vi "Scope_5772.vi"() -> ()   [LabVIEW 2013]
uses:
  <vilib>/rvi/interface/nirviReadWriteControl/nirviReadWriteControl.xnode
  <vilib>/rvi/errors/niLvFpgaAdjustHostInterfaceError.vi
  <vilib>/rvi/interface/nirviCloseFPGA/nirviCloseFPGA.xnode
  FPGA/DataMode.ctl
  <vilib>/rvi/interface/nirviOpenFPGA/nirviOpenFPGA.xnode
  <vilib>/Utility/error.llb/Error Cluster From Error Code.vi
  NiFpgaLv.dll
  <vilib>/rvi/interface/Simulation/niFpgaSimulationCallBeginRW.vi
  Host/Utilities/Ticker/Ticker.lvclass
  Host/Config/FPGAref.ctl
  Host/Scope/controls/ScopeMode.ctl
  FPGA Bitfiles/mixer_FPGATarget_FPGAmain5772_HJBBnI0CKw8.lvbitx
  <vilib>/FPGAPlugInAG/PXIe-7975R/niLvFpga_Open_PXIe-7975R.vi
  <vilib>/rvi/interface/common/dynamic/niFpgaDynamicAddResources.vi
  <vilib>/FPGAPlugInAG/Dynamic/niLvFpga_Close_Dynamic.vi
  <vilib>/userdefined/High Color/nirio_resource_hc.ctl
  <vilib>/Analysis/4window.llb/windowTd.ctl
  <vilib>/Analysis/NI_AALPro.lvlib
  Host/Scope/controls/power_spectrum_unit.ctl
panel:
  in  "Zoom freq X":bool
  in  "Zoom freq Y":bool
  in  "Zoom time Y":bool
  in  "Zoom time X":bool
  in  "Unit":T1
  in  "Window":T2=1 items=["Rectangle"=0, "Hanning"=1, "Hamming"=2, "Blackman-Harris"=3, "Exact Blackman"=4, "Blackman"=5, "Flat Top"=6, "4 Term B-Harris "=7, "7 Term B-Harris"=8, "Low Sidelobe"=9, "Blackman Nuttall"=11, "Triangle"=30, "Bartlett-Hanning"=31, "Bohman"=32, "Parzen"=33, "Welch"=34, "Kaiser"=60, "Dolph-Chebyshev"=61, "Gaussian"=62]
  in  "Samples to aqcuire":u32
  in  "Mode":T3
  in  "Mixer freq [MHz]":dbl
  in  "Phase offset (deg)":dbl
  in  "Fequency [MHz]":dbl
  in  "Ch1":bool
  in  "Ch0":bool
  out "freqdata":cluster{"f0":dbl, "df":dbl, "magnitude":dbl[]}[](graph)
  out "Timedata":dbl[][](graph)
  in  "Rumode":bool
  in  "Singleshot":bool
  in  "Ch1 Q":bool
  in  "Ch1 I":bool
  in  "Ch0 Q":bool
  in  "Ch0 I":bool
  out "error IO":errorcluster
  in  "stop":bool
  in  "resource name":T4="RIO0"
  out "Clocking Option Configured?":bool
  out "Configured?":bool
  # "Auto Zoom"
  # "Auto Zoom"
  # "FFT"
  # "Time domain"
  # "FPGA setup"
  # "Simulated data"
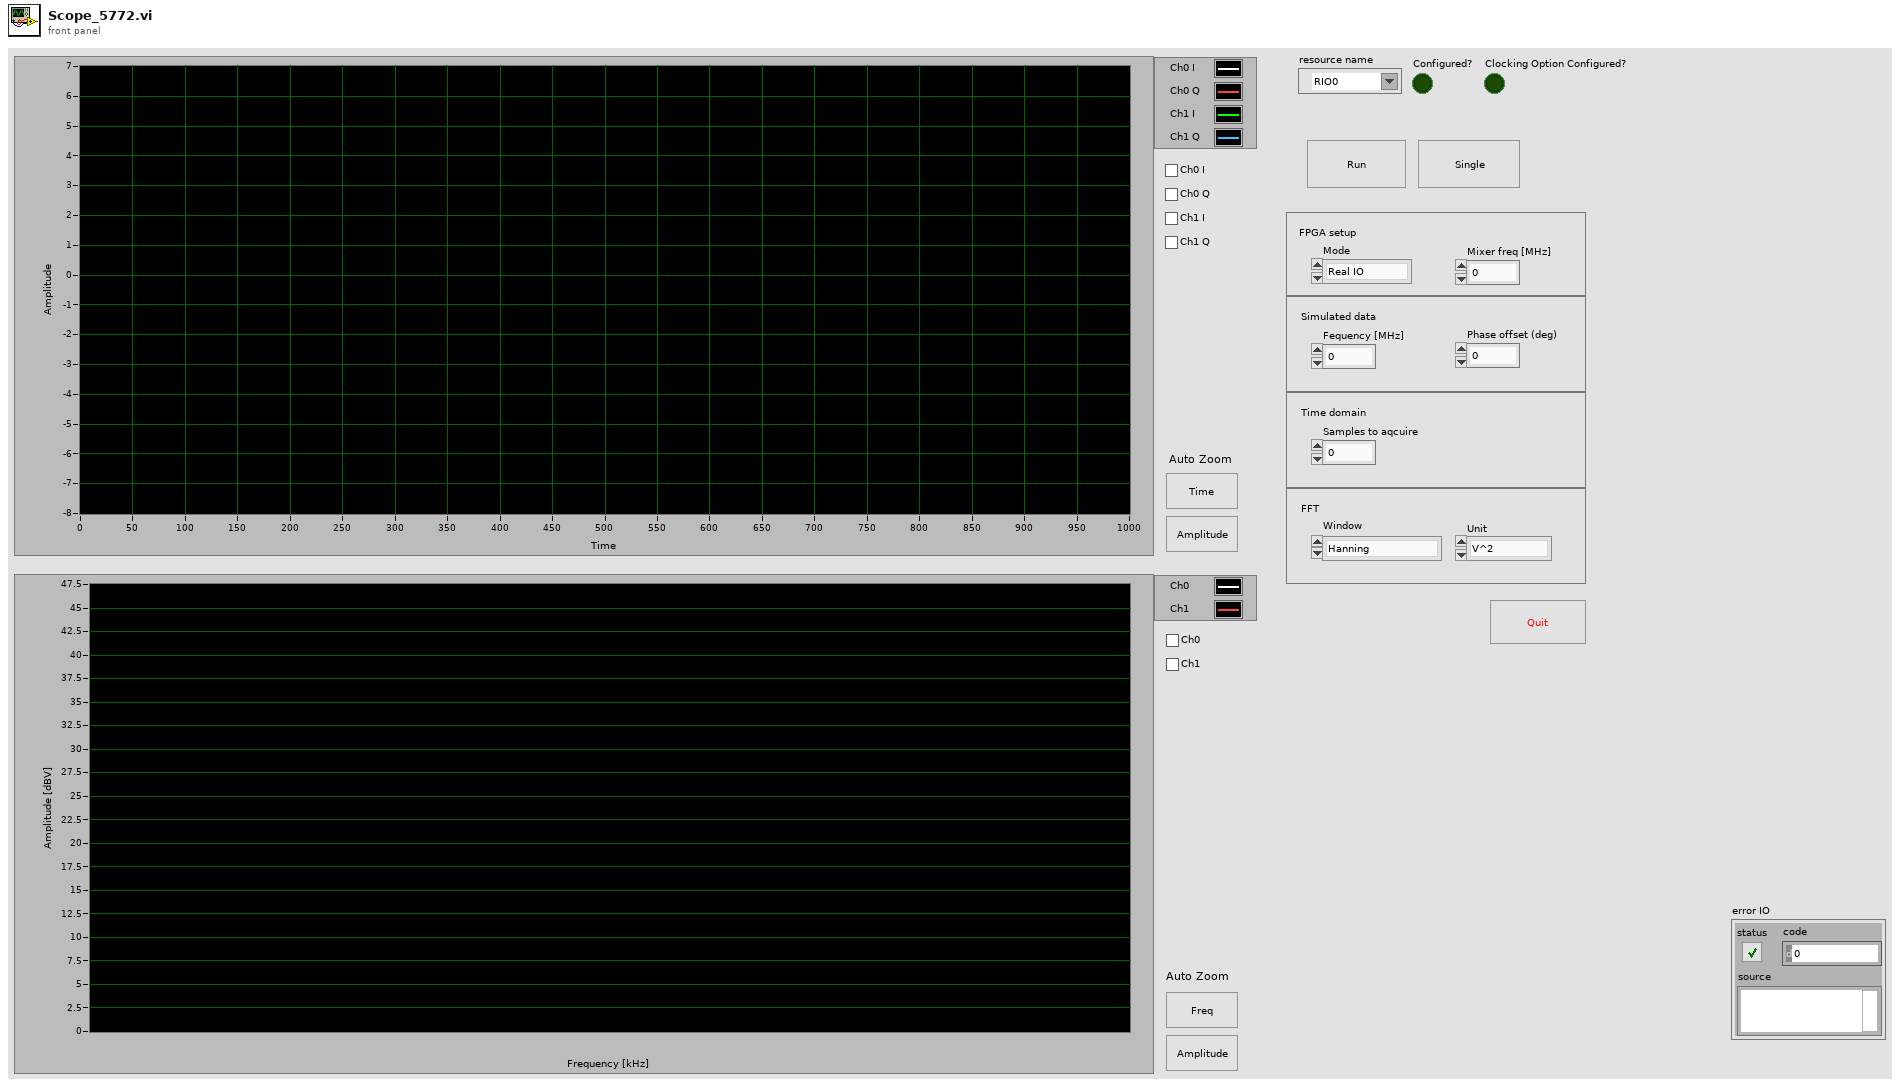
[diagram p1: front panel]
types:
  T1 = typedef "power_spectrum_unit.ctl" = enum16{"V^2", "V", "dBV"}
  T2 = typedef "NI_AALPro.lvlib/windowTd.ctl" = u32
  T3 = typedef "DataMode.ctl" = enum16{"Real IO", "Simulated"}
  T4 = typedef "nirio_resource_hc.ctl" = tag
  T5 = enum8{"Internal Clock PLL Off", "Internal Clock PLL On (REF IN)", "External Clock (CLK_IN)", "Internal Clock PLL On (IoModSyncClk)"}
  T6 = typedef "FPGAref.ctl" = refnum<k20>
  T7 = typedef "scope_params.ctl" = cluster{"scope mode":T8, "ticker":refnum<class "Ticker.lvclass">, "5160 samples per trigger":u32, "FPGA ref":T6, "P2P params":T9, "data mode":T3, "5782 samples per record":u32, "Chart length":i32}
  T8 = typedef "ScopeMode.ctl" = enum16{"Stopped", "Single", "Running", "Continuous"}
  T9 = typedef "P2P params.ctl" = cluster{"instrument handle":refnum<k15>, "stream session":refnum<k20>, "scale":cluster{"offset":dbl, "gain":dbl, "reserved 1":dbl, "reserved 2":dbl}, "actual sample rate":dbl, "Trigger":T10, "SCOPE Resource":refnum<k15>, "input impedance":u32}
  T10 = typedef "trigger_source.ctl" = enum16{"PFI 0", "PFI 1", "Software"}
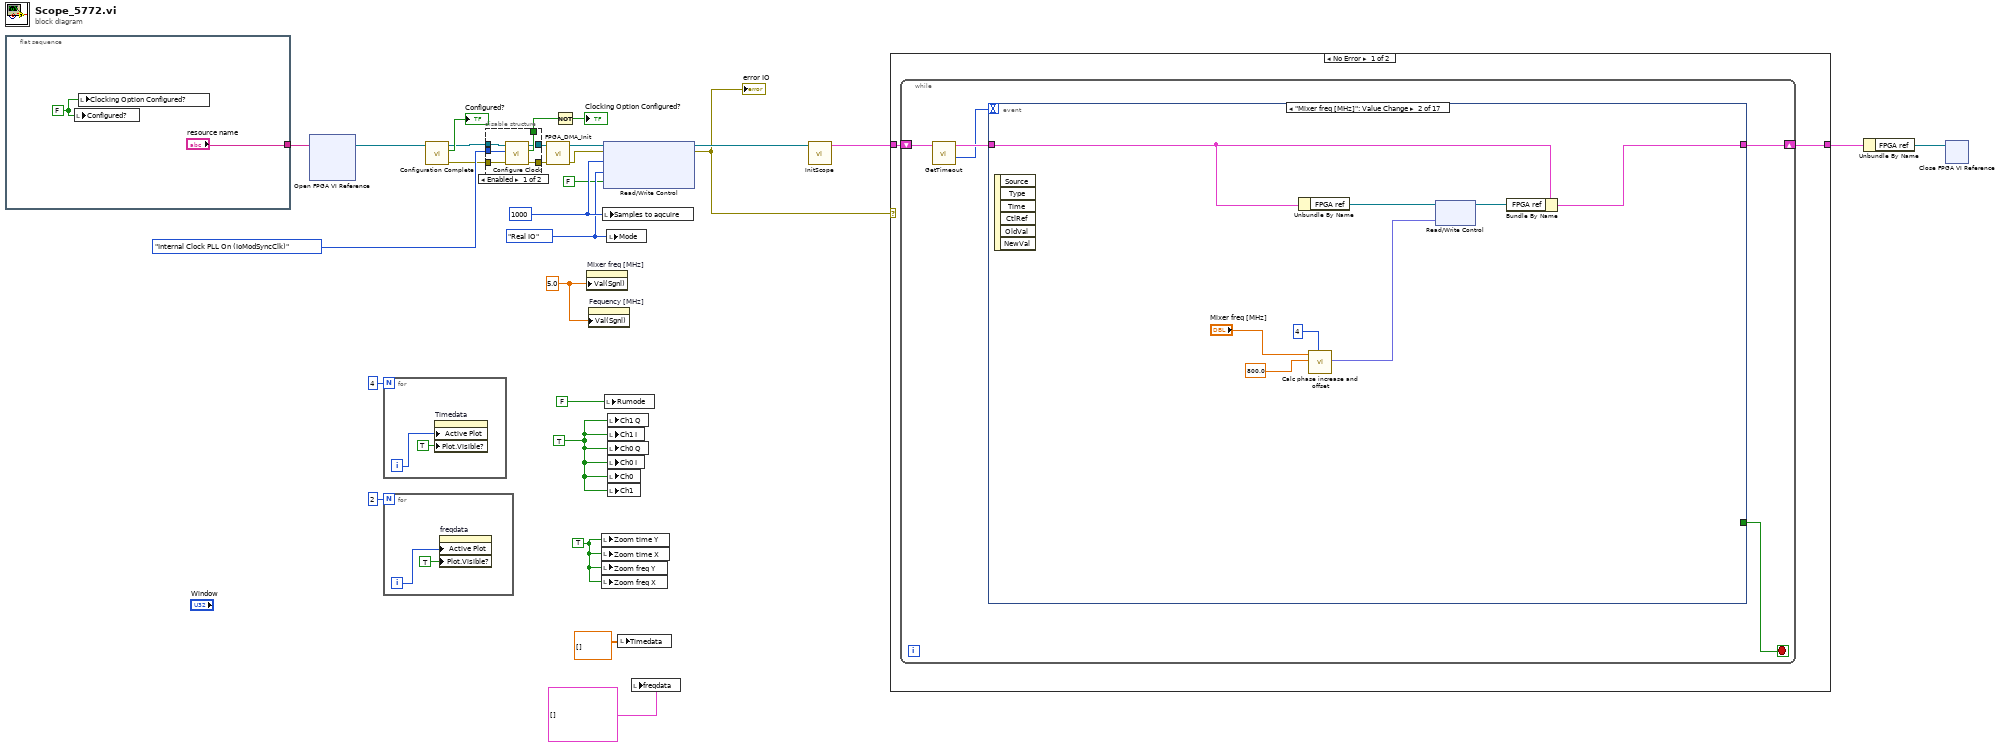
[diagram p0: block diagram]
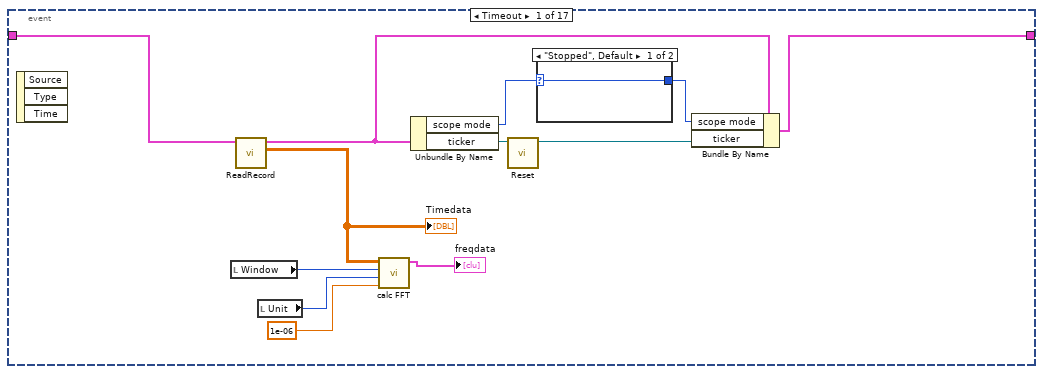
[diagram p3: hidden frame]
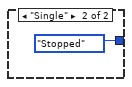
[diagram p4: hidden frame]
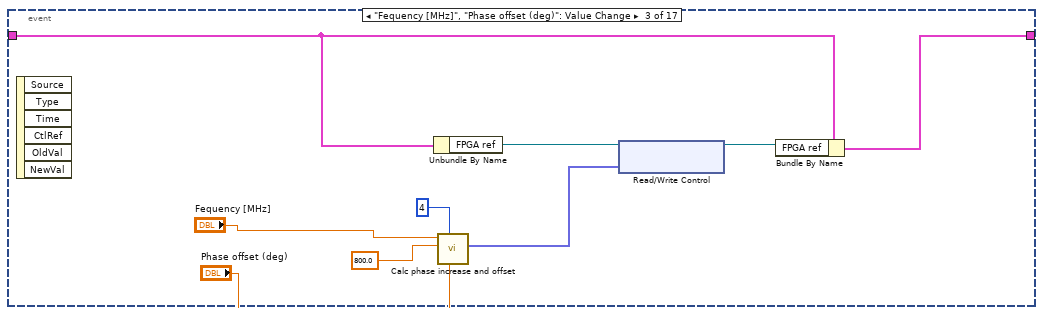
[diagram p5: hidden frame]
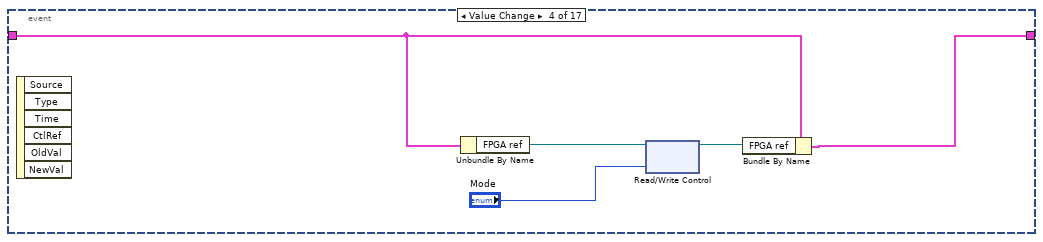
[diagram p6: hidden frame]
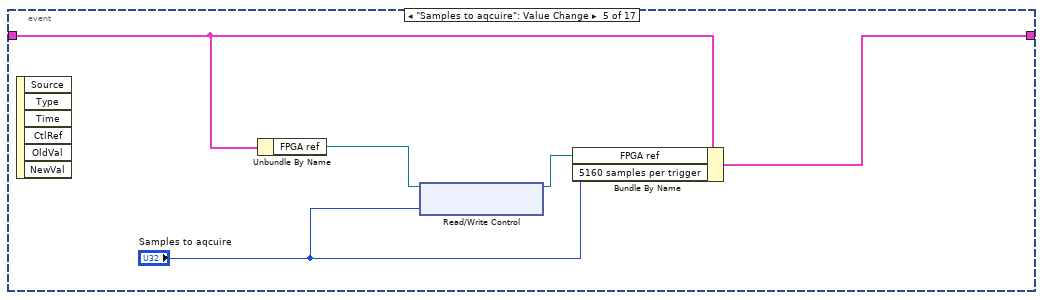
[diagram p7: hidden frame]
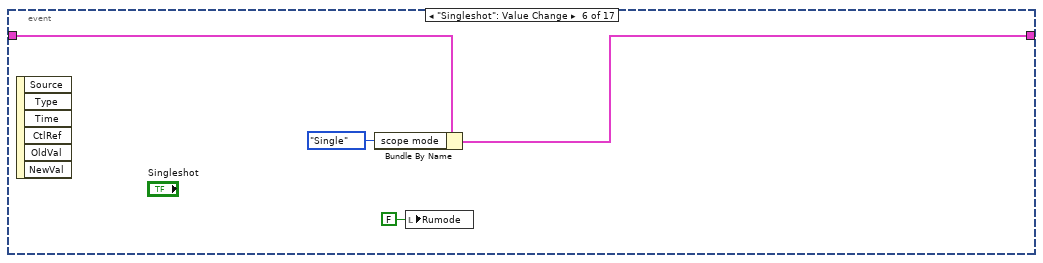
[diagram p8: hidden frame]
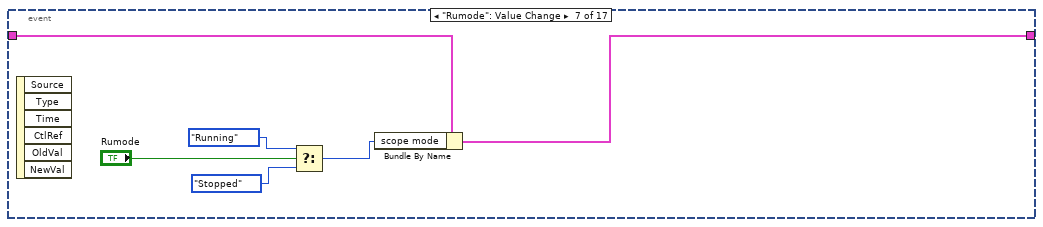
[diagram p9: hidden frame]
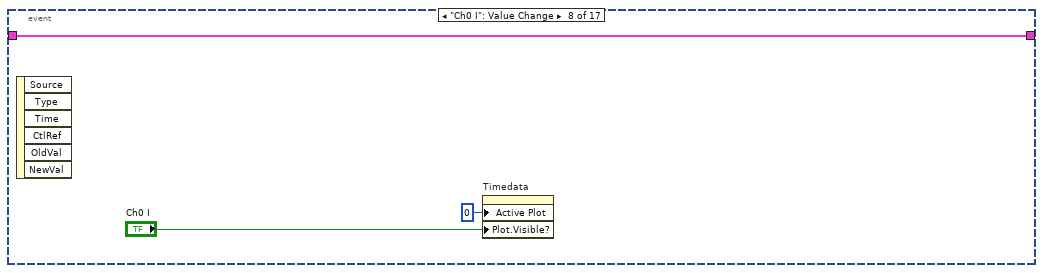
[diagram p10: hidden frame]
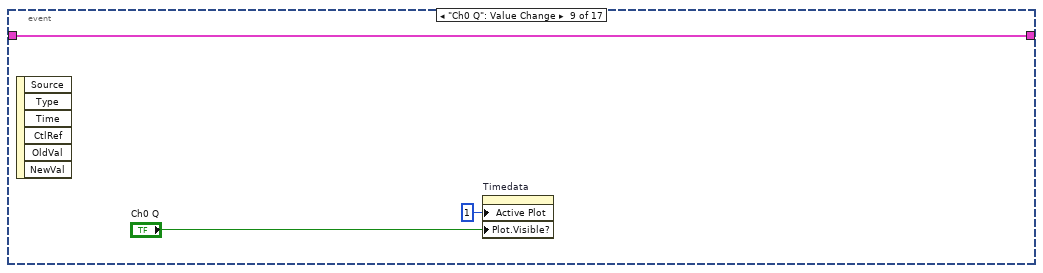
[diagram p11: hidden frame]
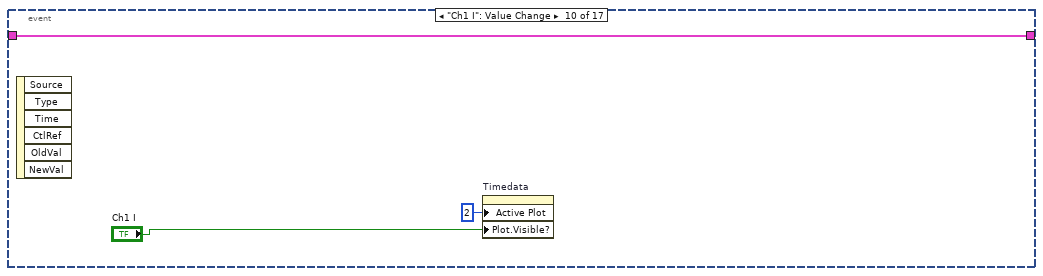
[diagram p12: hidden frame]
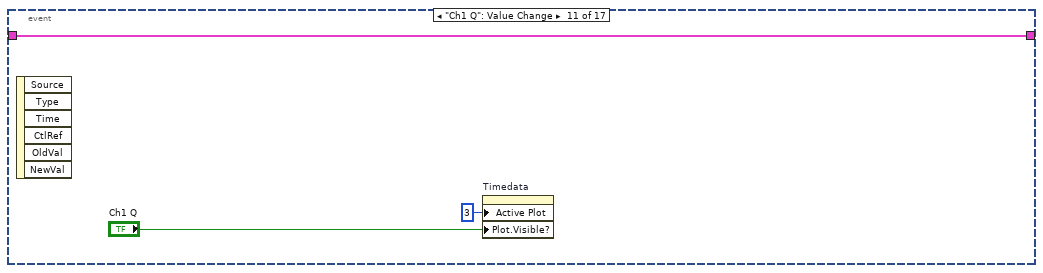
[diagram p13: hidden frame]
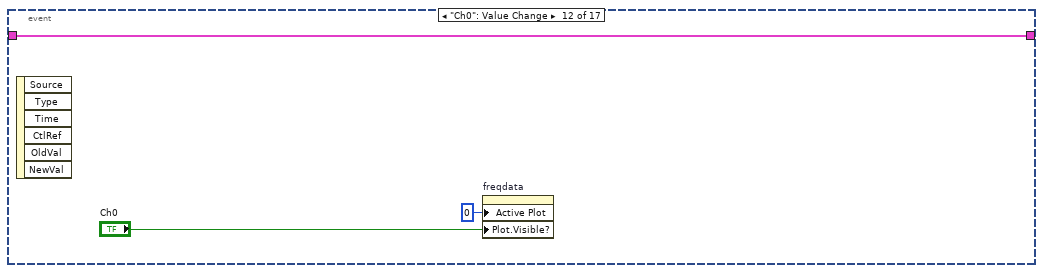
[diagram p14: hidden frame]
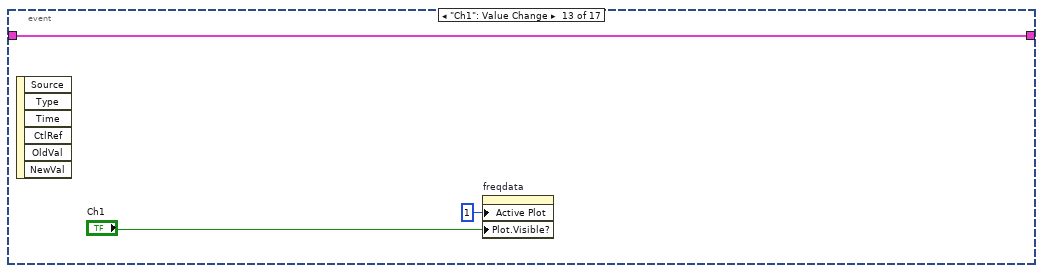
[diagram p15: hidden frame]
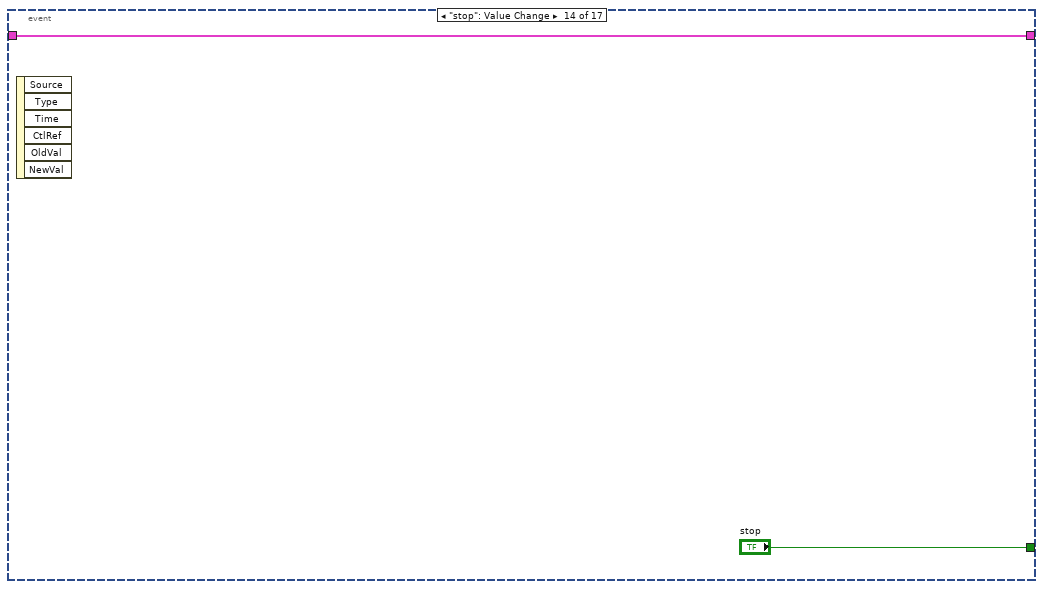
[diagram p16: hidden frame]
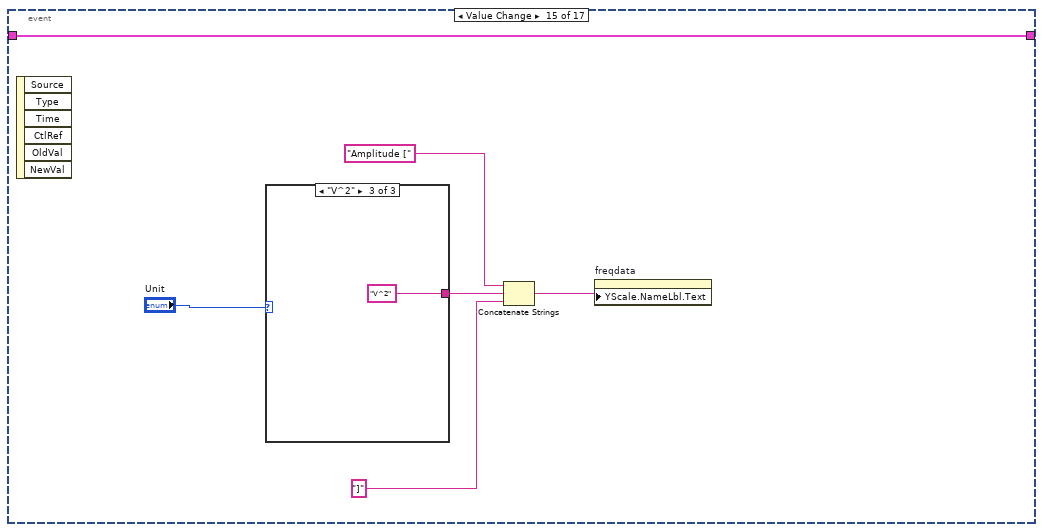
[diagram p17: hidden frame]
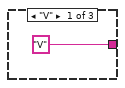
[diagram p18: hidden frame]
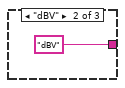
[diagram p19: hidden frame]
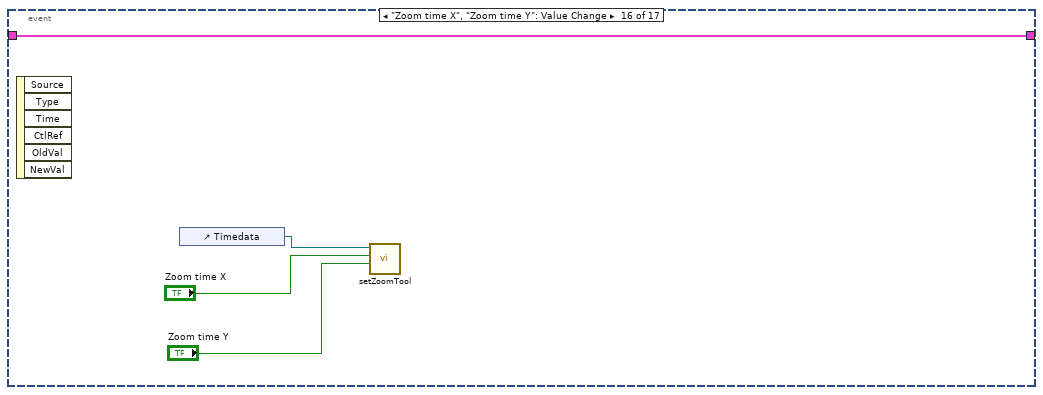
[diagram p20: hidden frame]
diagram:
  w1 = TRUE ("Rumode")
  w2 = TRUE ("Rumode")
  w6 = 5.0 ("Mixer requency [MHz]")
  w21 = DataMode."Real IO" ("Mode")
  w22 = u32 1000 ("Samples to aqcuire")
  n1 = flat-sequence {
    tunnel: ["resource name"] -> w16
    frame #0 {
      w29 = FALSE ("Trigger Acquisition")
      n2 = local write "Configured?"(w29) -> ()
      n3 = local write "Clocking Option Configured?"(w29) -> ()
    }
  }
  n4 = xnode "Open FPGA VI Reference"("resource name"=w16) -> ("FPGA VI Reference Out"=w11:refnum<k20>)  [unwired: 1 in, 1 out]
  n5 = for {
    N: 4 -> [_]
    i -> [w32]
    n6 = property on="Timedata" class="WFGraph (strict)"("Active Plot"=w32, "Plot.Visible?"=TRUE ("Plot.Visible")) -> ()  [unwired: 2 in, 2 out]
  }
  n7 = for {
    N: 2 -> [_]
    i -> [w33]
    n8 = property on="freqdata" class="WFGraph (strict)"("Active Plot"=w33, "Plot.Visible?"=TRUE ("Plot.Visible")) -> ()  [unwired: 2 in, 2 out]
  }
  n9 = call "Configuration Complete.vi"("FPGA VI Reference in"=w11) -> ("error out"=w19:errorcluster, "Configured?"=→"Configured?":bool, "FPGA VI Reference Out"=w9:T6)  [unwired: 8 in]
  n10 = disable-structure shown="Enabled" {
    disable-tunnel: [w40 _] -> w26
    disable-tunnel: T5."Internal Clock PLL On (IoModSyncClk)" ("Clock Source") -> [w39 _]
    disable-tunnel: [w38 w42] -> w24
    disable-tunnel: w19 -> [w37 w41]
    disable-tunnel: [w36 w41] -> w18
    disable-tunnel: w9 -> [w35 _]
    frame Enabled {
      n11 = call "Configure Clock.vi"("error in"=w37, "Clock Source"=w39, "FPGA VI Reference in"=w35) -> ("error out"=w36:errorcluster, "Configuration Error"=w40:bool, "FPGA VI Reference Out"=w38:T6)  [unwired: 6 in]
    }
    frame Disabled {
    }
  }
  n12 = call "FPGA_DMA_Init.vi"("error in (no error)"=w18, "FPGA VI Reference"=w24) -> ("error out"=w17:errorcluster, "FPGA VI out"=w23:T6)  [unwired: 7 in, 1 out]
  n13 = Not(x=w26) -> (.not. x?=→"Clocking Option Configured?":bool)
  n14 = property on="Mixer freq [MHz]" class="DigNum (strict)"("Val(Sgnl)"=w6) -> ()  [unwired: 2 in, 2 out]
  n15 = property on="Fequency [MHz]" class="DigNum (strict)"("Val(Sgnl)"=w6) -> ()  [unwired: 2 in, 2 out]
  n16 = local write "Zoom time Y"(w1) -> ()
  n17 = local write "Zoom time X"(w1) -> ()
  n18 = local write "Zoom freq Y"(w1) -> ()
  n19 = local write "Zoom freq X"(w1) -> ()
  n20 = local write "Samples to aqcuire"(w22) -> ()
  n21 = xnode "Read/Write Control"("FPGA VI Reference In"=w23, "error in"=w17, "Samples Per Trigger"=w22, "Mode"=w21, "Trigger Acquisition"=FALSE) -> ("FPGA VI Reference Out"=w12:T6, "error out"=w10:errorcluster)
  "error IO" <- w10
  n22 = local write "Rumode"(FALSE ("Rumode")) -> ()
  n23 = local write "Mode"(w21) -> ()
  n24 = local write "Ch1 Q"(w2) -> ()
  n25 = local write "Ch1 I"(w2) -> ()
  n26 = local write "Ch0 Q"(w2) -> ()
  n27 = local write "Ch0 I"(w2) -> ()
  n28 = local write "Ch0"(w2) -> ()
  n29 = local write "Ch1"(w2) -> ()
  n30 = local write "Timedata"(dbl[][] [] ("Timedata")) -> ()
  n31 = local write "freqdata"(cluster{"f0":dbl, "df":dbl, "magnitude":dbl[]}[] [] ("freqdata")) -> ()
  n32 = call "InitScope.vi"("FPGA VI Reference"=w12) -> ("scope params"=w15:T7)  [unwired: 10 in]
  n33 = case shown="No Error" w10 {
    tunnel: w15 -> [w44 w138]
    tunnel: [w43 w138] -> w14
    frame No Error {
      n34 = while {
        shift-right: [w48] -> w43
        shift-left: w44 -> [w47]
        stop <- w49 stop-if-true
        n35 = call "GetTimeout.vi"("scope in"=w47) -> ("Time left"=w45:i32, "scope out"=w46:T7)  [unwired: 9 in]
        n36 = event shown="[1] \"Mixer freq [MHz]\": Value Change" {
          selector: _ -> [_ _ _ _ _ _ _ _ _ _ _ _ _ _ _ _ _]
          dyn-events: _ -> [_ _ _ _ _ _ _ _ _ _ _ _ _ _ _ _ _]
          timeout: w45 -> [_ _ _ _ _ _ _ _ _ _ _ _ _ _ _ _ _]
          tunnel: [_ _ _ _ _ _ _ _ _ _ _ _ _ "stop" _ _ _] -> w49
          tunnel: w46 -> [w61 w66 w76 w83 w87 w93 w100 w103 w106 w109 w112 w115 w118 w119 w126 w133 w137]
          tunnel: [w57 w64 w75 w82 w86 w92 w99 w103 w106 w109 w112 w115 w118 w119 w126 w133 w137] -> w48
          event Timeout {
            n37 = event-data() -> ()  [unwired: 1 in, 3 out]
            n38 = local read "Window"() -> (w52:T2)
            n39 = call "ReadRecord.vi"("scope params"=w61) -> ("data"=w54:dbl[][], "scope params out"=w58:T7)  [unwired: 8 in, 1 out]
            "Timedata" <- w54
            n40 = local read "Unit"() -> (w51:T1)
            n41 = call "calc FFT.vi"("dt"=1e-06, "Unit"=w51, "Window"=w52, "data"=w54) -> ("Power Spectrum / PSD"=→"freqdata":cluster{"f0":dbl, "df":dbl, "magnitude":dbl[]}[])  [unwired: 7 in]
            n42 = Unbundle By Name(w58) -> ("scope mode"=w56:T8, "ticker"=w60:refnum<class "Ticker.lvclass">)
            n43 = call "Reset.vi"("Ticker in"=w60) -> ("Ticker out"=w59:refnum<class "Ticker.lvclass">)  [unwired: 9 in, 1 out]
            n44 = case shown="\"Stopped\", Default" w56 {
              selector: w56 -> [w62 _]
              tunnel: [w62 ScopeMode."Stopped" ("scope mode")] -> w55
              frame "Stopped", Default {
              }
              frame "Single" {
              }
            }
            n45 = Bundle By Name(cluster=w58, "scope mode"=w55, "ticker"=w59) -> (w57:T7)
          }
          event "Mixer freq [MHz]": Value Change {
            n46 = event-data() -> ()  [unwired: 1 in, 6 out]
            n47 = Unbundle By Name(w66) -> ("FPGA ref"=w67:T6)
            n48 = call "Calc phase increase and offset.vi"("# of DDS"=4, "fclk (MHz)"=800.0 ("fclk (800MHz)"), "f_generated (MHz)"="Mixer freq [MHz]") -> ("Phase out"=w69:fxp<+,64,64>[])  [unwired: 6 in, 2 out]
            n49 = xnode "Read/Write Control"("FPGA VI Reference In"=w67, "Phase"=w69) -> ("FPGA VI Reference Out"=w65:T6)  [unwired: 1 in, 1 out]
            n50 = Bundle By Name(cluster=w66, "FPGA ref"=w65) -> (w64:T7)
          }
          event "Fequency [MHz]", "Phase offset (deg)": Value Change {
            n51 = event-data() -> ()  [unwired: 1 in, 6 out]
            n52 = Unbundle By Name(w76) -> ("FPGA ref"=w78:T6)
            n53 = call "Calc phase increase and offset.vi"("Phase offset (deg)"="Phase offset (deg)", "# of DDS"=4, "fclk (MHz)"=800.0 ("fclk (800MHz)"), "f_generated (MHz)"="Fequency [MHz]") -> ("Phase out"=w72:fxp<+,64,64>[])  [unwired: 5 in, 2 out]
            n54 = xnode "Read/Write Control"("FPGA VI Reference In"=w78, "Simulated phase"=w72) -> ("FPGA VI Reference Out"=w77:T6)  [unwired: 1 in, 1 out]
            n55 = Bundle By Name(cluster=w76, "FPGA ref"=w77) -> (w75:T7)
          }
          event Value Change {
            n56 = event-data() -> ()  [unwired: 1 in, 6 out]
            n57 = Unbundle By Name(w83) -> ("FPGA ref"=w85:T6)
            n58 = xnode "Read/Write Control"("FPGA VI Reference In"=w85, "Mode"="Mode") -> ("FPGA VI Reference Out"=w84:T6)  [unwired: 1 in, 1 out]
            n59 = Bundle By Name(cluster=w83, "FPGA ref"=w84) -> (w82:T7)
          }
          event "Samples to aqcuire": Value Change {
            n60 = event-data() -> ()  [unwired: 1 in, 6 out]
            n61 = Unbundle By Name(w87) -> ("FPGA ref"=w90:T6)
            n62 = xnode "Read/Write Control"("FPGA VI Reference In"=w90, "Samples Per Trigger"="Samples to aqcuire") -> ("FPGA VI Reference Out"=w89:T6)  [unwired: 1 in, 1 out]
            n63 = Bundle By Name(cluster=w87, "FPGA ref"=w89, "5160 samples per trigger"="Samples to aqcuire") -> (w86:T7)
          }
          event "Singleshot": Value Change {
            n64 = event-data() -> ()  [unwired: 1 in, 6 out]
            n65 = Bundle By Name(cluster=w93, "scope mode"=ScopeMode."Single") -> (w92:T7)
            n66 = local write "Rumode"(FALSE ("Rumode")) -> ()
          }
          event "Rumode": Value Change {
            n67 = event-data() -> ()  [unwired: 1 in, 6 out]
            n68 = Select(t=ScopeMode."Running" ("scope mode"), s="Rumode", f=ScopeMode."Stopped" ("scope mode")) -> (s? t:f=w95:T8)
            n69 = Bundle By Name(cluster=w100, "scope mode"=w95) -> (w99:T7)
          }
          event "Ch0 I": Value Change {
            n70 = event-data() -> ()  [unwired: 1 in, 6 out]
            n71 = property on="Timedata" class="WFGraph (strict)"("Active Plot"=u32 0, "Plot.Visible?"="Ch0 I") -> ()  [unwired: 2 in, 2 out]
          }
          event "Ch0 Q": Value Change {
            n72 = event-data() -> ()  [unwired: 1 in, 6 out]
            n73 = property on="Timedata" class="WFGraph (strict)"("Active Plot"=u32 1, "Plot.Visible?"="Ch0 Q") -> ()  [unwired: 2 in, 2 out]
          }
          event "Ch1 I": Value Change {
            n74 = event-data() -> ()  [unwired: 1 in, 6 out]
            n75 = property on="Timedata" class="WFGraph (strict)"("Active Plot"=u32 2, "Plot.Visible?"="Ch1 I") -> ()  [unwired: 2 in, 2 out]
          }
          event "Ch1 Q": Value Change {
            n76 = event-data() -> ()  [unwired: 1 in, 6 out]
            n77 = property on="Timedata" class="WFGraph (strict)"("Active Plot"=u32 3, "Plot.Visible?"="Ch1 Q") -> ()  [unwired: 2 in, 2 out]
          }
          event "Ch0": Value Change {
            n78 = event-data() -> ()  [unwired: 1 in, 6 out]
            n79 = property on="freqdata" class="WFGraph (strict)"("Active Plot"=u32 0, "Plot.Visible?"="Ch0") -> ()  [unwired: 2 in, 2 out]
          }
          event "Ch1": Value Change {
            n80 = event-data() -> ()  [unwired: 1 in, 6 out]
            n81 = property on="freqdata" class="WFGraph (strict)"("Active Plot"=u32 1, "Plot.Visible?"="Ch1") -> ()  [unwired: 2 in, 2 out]
          }
          event "stop": Value Change {
            n82 = event-data() -> ()  [unwired: 1 in, 6 out]
          }
          event Value Change {
            n83 = event-data() -> ()  [unwired: 1 in, 6 out]
            n84 = case shown="\"V^2\"" "Unit" {
              tunnel: ["V" "dBV" "V^2"] -> w123
              frame "V" {
              }
              frame "dBV" {
              }
              frame "V^2" {
              }
            }
            n85 = Concatenate Strings("Amplitude [", w123, "]") -> (w121:string)
            n86 = property on="freqdata" class="WFGraph (strict)"("YScale.NameLbl.Text"=w121) -> ()  [unwired: 2 in, 2 out]
          }
          event "Zoom time X", "Zoom time Y": Value Change {
            n87 = event-data() -> ()  [unwired: 1 in, 6 out]
            n88 = control-ref of="Timedata"() -> (w132:refnum<vi>)
            n89 = call "setZoomTool.vi"("Zoom Y"="Zoom time Y", "Zoom  X"="Zoom time X", "reference"=w132) -> ()  [unwired: 9 in]
          }
          event "Zoom freq Y", "Zoom freq X": Value Change {
            n90 = event-data() -> ()  [unwired: 1 in, 6 out]
            n91 = control-ref of="freqdata"() -> (w134:refnum<vi>)
            n92 = call "setZoomTool.vi"("Zoom Y"="Zoom freq Y", "Zoom  X"="Zoom freq X", "reference"=w134) -> ()  [unwired: 9 in]
          }
        }
      }
    }
    frame Error {
    }
  }
  n93 = Unbundle By Name(w14) -> ("FPGA ref"=w13:T6)
  n94 = xnode "Close FPGA VI Reference"("FPGA VI Reference In"=w13) -> ()  [unwired: 1 in, 1 out]
